vi "Compile Datalog Array.vi"() -> ()   [LabVIEW 2017]
uses:
  Y Axis Motor Cluster.ctl
  X Axis Motor Cluster.ctl
  <vilib>/myRIO/Common/Instrument Driver Framework/myRIO v1.0/Encoder/typedefs/Encoder Count Direction Enum.ctl
  Encoder Cluster.ctl
  Coords Input Cluster.ctl
panel:
  out "Data Array":dbl[][](array[numeric])
  in  "Coordinates Input":T1
  in  "Total Runtime (s)":dbl format="%.2f"
  in  "Loop Runtime (s)":dbl format="%.3f"
  in  "Encoder Output":T2
  in  "X Axis Motor Params":T4
  in  "Y Axis Motor Params":T5
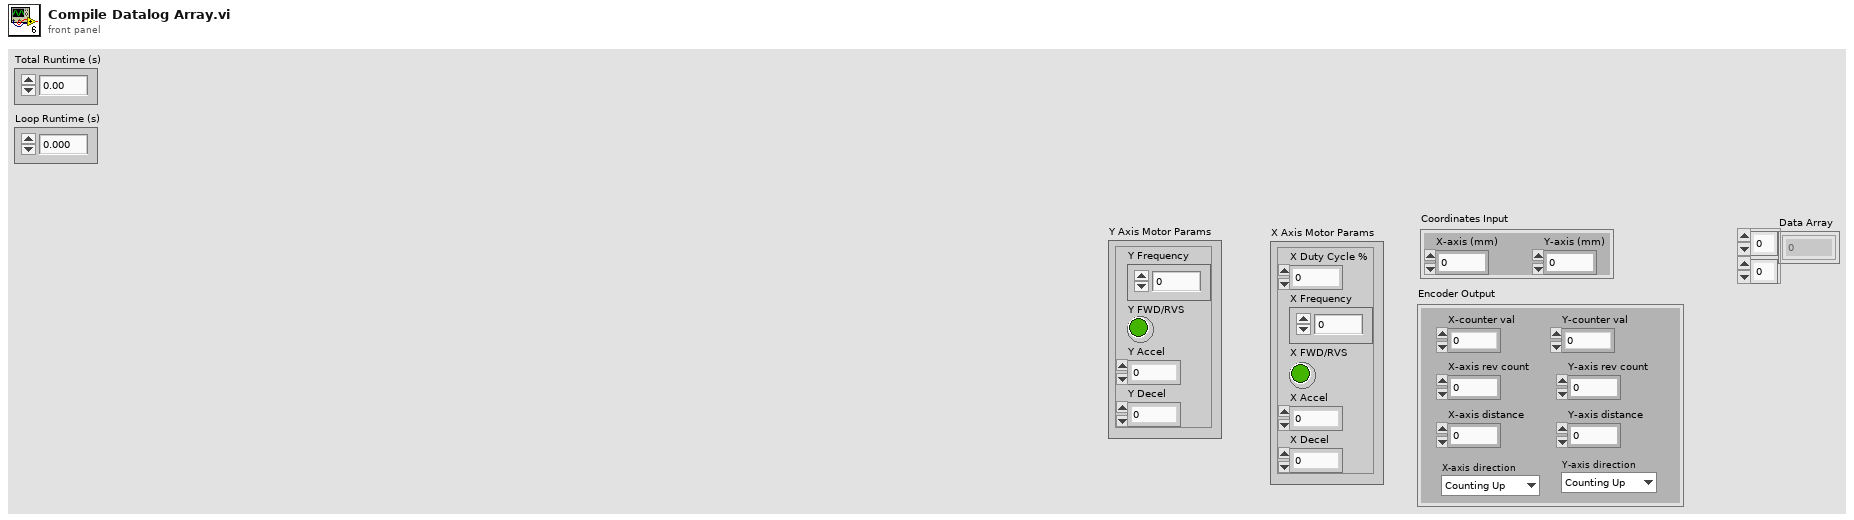
[diagram p1: front panel]
types:
  T1 = typedef "Coords Input Cluster.ctl" = cluster{"X-axis (mm)":dbl, "Y-axis (mm)":dbl}
  T2 = typedef "Encoder Cluster.ctl" = cluster{"Y-axis rev count":dbl, "Y-axis distance":dbl, "X-axis rev count":dbl, "X-axis distance":dbl, "Y-axis direction":T3, "X-axis direction":T3, "X-counter val":i32, "Y-counter val":i32}
  T3 = typedef "Encoder Count Direction Enum.ctl" = enum16{"Counting Up", "Counting Down"}
  T4 = typedef "X Axis Motor Cluster.ctl" = cluster{"X Frequency":dbl, "X FWD/RVS":bool, "X Accel":dbl, "X Decel":dbl, "X Duty Cycle %":dbl}
  T5 = typedef "Y Axis Motor Cluster.ctl" = cluster{"Y Frequency":dbl, "Y FWD/RVS":bool, "Y Accel":dbl, "Y Decel":dbl}
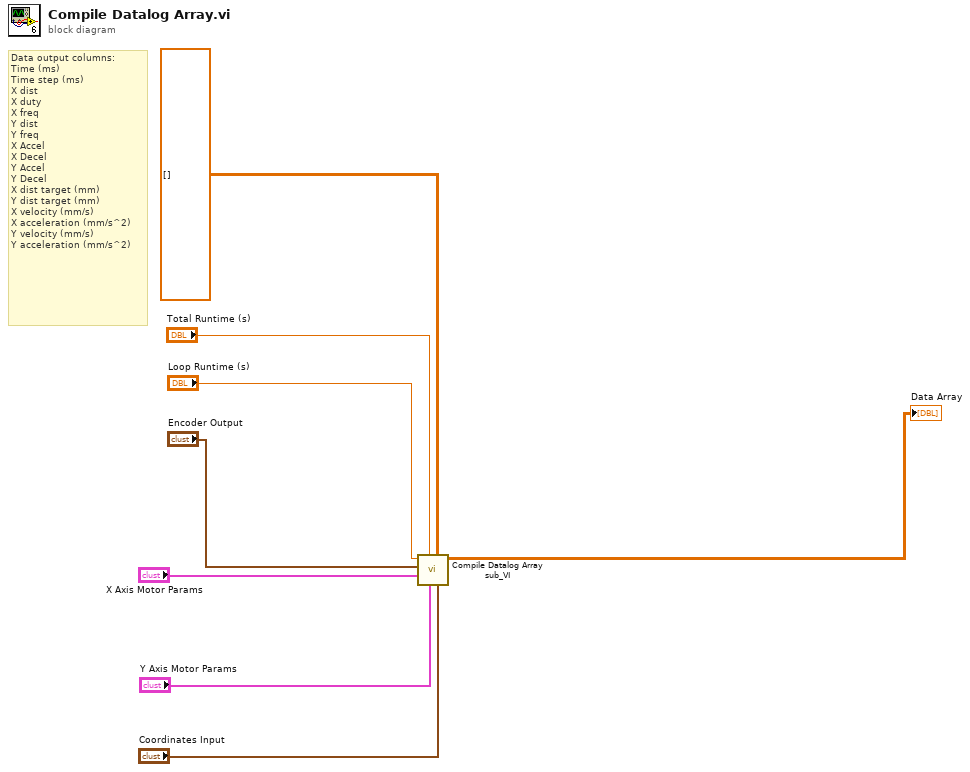
[diagram p0: block diagram]
diagram:
  # "Data output columns:\nTime (ms)\nTime step (ms)\nX dist\nX duty\nX freq\nY dist\nY freq\nX Accel\nX Decel\nY Accel\nY Decel\nX dist target (mm)\nY dist target (mm)\nX velocity (mm/s)\nX acceleration (mm/s^2)\nY velocity (mm/s)\nY acceleration (mm/s^2)"
  n1 = call "Compile Datalog Array sub_VI.vi"("Coordinates Input"="Coordinates Input", "Array in"=dbl[][] [], "Y Axis Motor Params"="Y Axis Motor Params", "Total Runtime (s)"="Total Runtime (s)", "X Axis Motor Params"="X Axis Motor Params", "Encoder Output"="Encoder Output", "Loop Runtime (s)"="Loop Runtime (s)") -> ("Array out"=→"Data Array":dbl[][])  [unwired: 4 in]
